vi "Destroy Data Channels.vi"(8 "error in":errorcluster, 11 "Node in":refnum<class "AMS Power Supply Template.lvclass">) -> (0 "error out":errorcluster, 3 "Node out":refnum<class "AMS Power Supply Template.lvclass">)   [LabVIEW 2023, in "AMS Power Supply Template.lvlib" / "AMS Power Supply Template.lvclass"]
uses:
  AMS Power Supply Template.lvclass
  AMS Power Supply Template.lvclass/AMS Power Supply Template.ctl
  Capabilities/Capabilities/High Level Capabilities/Power Supply/Power Supply.lvclass
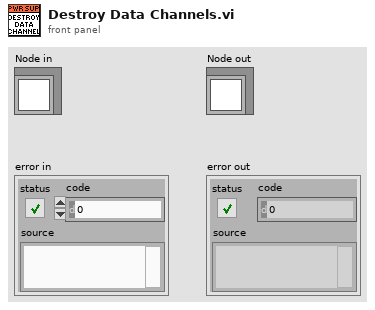
[diagram p1: front panel]
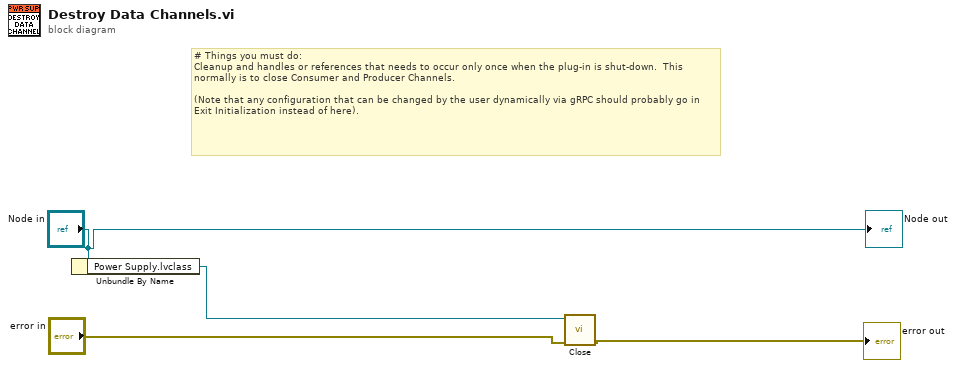
[diagram p0: block diagram]
diagram:
  # "# Things you must do:\nCleanup and handles or references that needs to occur only once when the plug-in is shut-down.  This normally is to close Consumer and Producer Channels.   \n\n(Note that any configuration that can be changed by the user dynamically via gRPC should probably go in Exit Initialization instead of here)."
  n1 = Unbundle By Name("Node in") -> ("Power Supply.lvclass"=w4:refnum<class "Power Supply.lvclass">)
  n2 = call-dynamic "Close.vi"("error in"="error in", "Power Supply In"=w4) -> ("error out"=→"error out":errorcluster)  [unwired: 8 in, 1 out]
  "Node out" <- "Node in"
